vi "Alpha Mask.vi"(5 "State":enum16{"Init", "Open", "Close"}(ring)=enum."Close", 8 "error in (no error)":errorcluster, 10 "This VI":refnum<vi>, 11 "Button Ref":refnum<vi>) -> (0 "error out":errorcluster, 2 "Position Output":cluster{i16, i16})   [LabVIEW 2020, in "Popup Dialog.lvlib"]
uses:
  Popup Dialog.lvlib
  <vilib>/Utility/miscctls.llb/LVPositionTypeDef.ctl
panel:
  # "References"
  # "Errors"
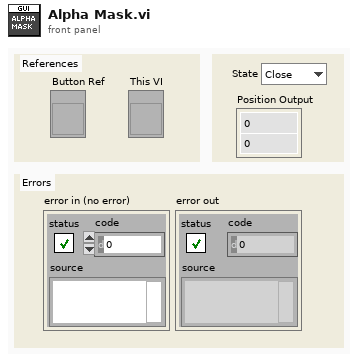
[diagram p1: front panel]
types:
  T1 = typedef "LVPositionTypeDef.ctl" = cluster{"Left":i32, "Top":i32}
  T2 = typedef "LVRectTypeDef.ctl" = cluster{"Left":i16, "Top":i16, "Right":i16, "Bottom":i16}
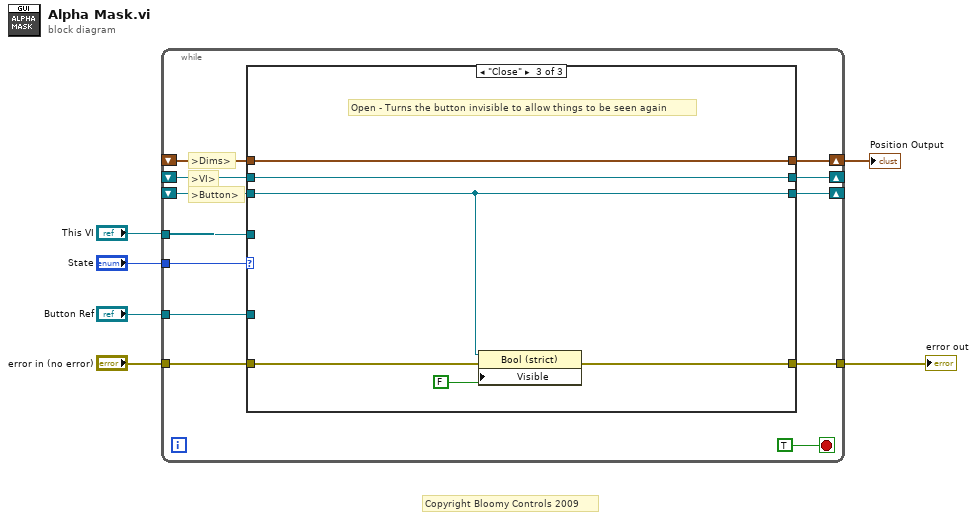
[diagram p0: block diagram]
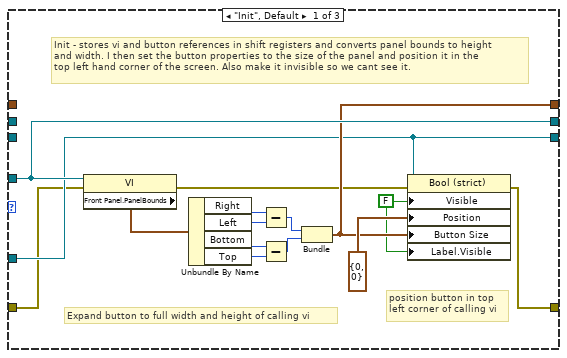
[diagram p2: hidden frame]
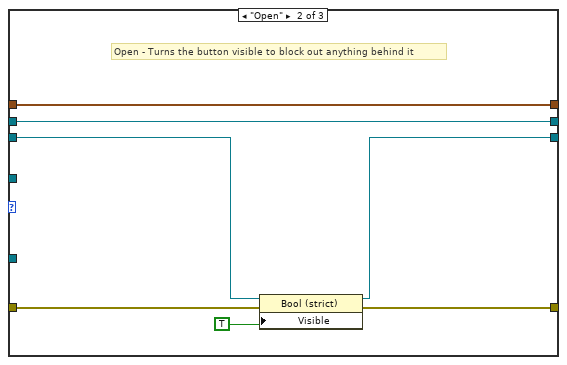
[diagram p3: hidden frame]
diagram:
  # "Copyright Bloomy Controls 2009"
  n1 = while {
    tunnel: "This VI" -> [w18]
    tunnel: "State" -> [w17]
    shift-right: [w16] -> w3
    shift-left: _ -> [w10]
    shift-right: [w15] -> _
    shift-left: _ -> [w11]
    tunnel: "Button Ref" -> [w13]
    shift-right: [w14] -> _
    shift-left: _ -> [w12]
    tunnel: [w8] -> w2
    tunnel: "error in (no error)" -> [w7]
    stop <- TRUE stop-if-true
    # ">Button>"
    # ">VI>"
    # ">Dims>"
    n2 = case shown="\"Close\"" w17 {
      tunnel: w18 -> [w30 _ _]
      tunnel: [w28 w36 w43] -> w16
      tunnel: [w30 w37 w44] -> w15
      tunnel: [w27 w38 w45] -> w14
      tunnel: w13 -> [w27 _ _]
      tunnel: w12 -> [_ w39 w45]
      tunnel: w11 -> [_ w37 w44]
      tunnel: w10 -> [_ w36 w43]
      tunnel: [w24 w34 w42] -> w8
      tunnel: w7 -> [w26 w35 w41]
      frame "Init", Default {
        w19 = FALSE ("Visible")
        # "Init - stores vi and button references in shift registers and converts panel bounds to height\nand width. I then set the button properties to the size of the panel and position it in the\ntop left hand corner of the screen. Also make it invisible so we cant see it."
        # "position button in top\nleft corner of calling vi"
        # "Expand button to full width and height of calling vi"
        n3 = property class="VI"(reference=w30, error in=w26) -> (error out=w25:errorcluster, "Front Panel.PanelBounds"=w31:T2)  [unwired: 1 out]
        n4 = Unbundle By Name(w31) -> ("Right"=w23:i16, "Left"=w22:i16, "Bottom"=w21:i16, "Top"=w20:i16)
        n5 = Subtract(x=w23, y=w22) -> (x-y=w32:i16)
        n6 = Subtract(x=w21, y=w20) -> (x-y=w33:i16)
        n7 = Bundle(w32, w33) -> (w28:cluster{i16, i16})  [unwired: 1 out]
        n8 = property on="Property Node" class="Bool (strict)"(reference=w27, error in=w25, "Visible"=w19, "Position"=T1 {"Left"=0, "Top"=0}, "Button Size"=w28, "Label.Visible"=w19) -> (error out=w24:errorcluster)  [unwired: 1 out]
      }
      frame "Open" {
        # "Open - Turns the button visible to block out anything behind it"
        n9 = property on="Property Node" class="Bool (strict)"(reference=w39, error in=w35, "Visible"=TRUE) -> (reference out=w38:refnum<vi>, error out=w34:errorcluster)
      }
      frame "Close" {
        # "Open - Turns the button invisible to allow things to be seen again"
        n10 = property on="Property Node" class="Bool (strict)"(reference=w45, error in=w41, "Visible"=FALSE) -> (error out=w42:errorcluster)  [unwired: 1 out]
      }
    }
  }
  "Position Output" <- w3
  "error out" <- w2
